vi "Collect Data2D.vi"(8 "error in (no error)":errorcluster, 10 "Data2D in":refnum<class "Data2D.lvclass">, 11 "AbstractCollector2D in":refnum<class "AbstractCollector2D.lvclass">) -> (0 "error out":errorcluster, 2 "finished?":bool=TRUE, 3 "AbstractCollector2D out":refnum<class "AbstractCollector2D.lvclass">)   [LabVIEW 2014, in "AbstractCollector2D.lvclass"]
uses:
  AbstractCollector2D.lvclass
  Model/Data/Data2D/Data2D.lvclass
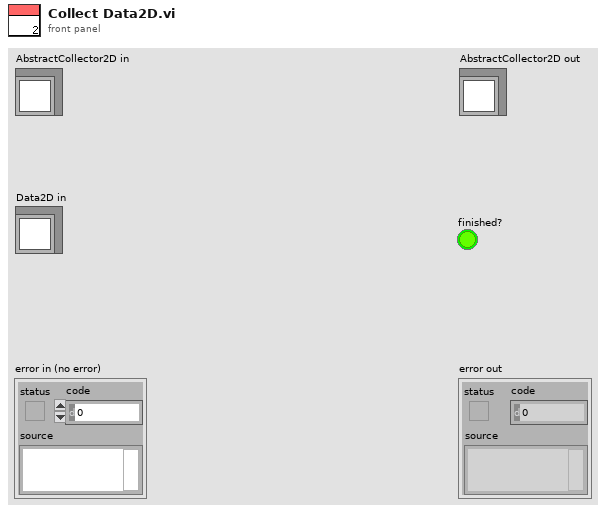
[diagram p1: front panel]
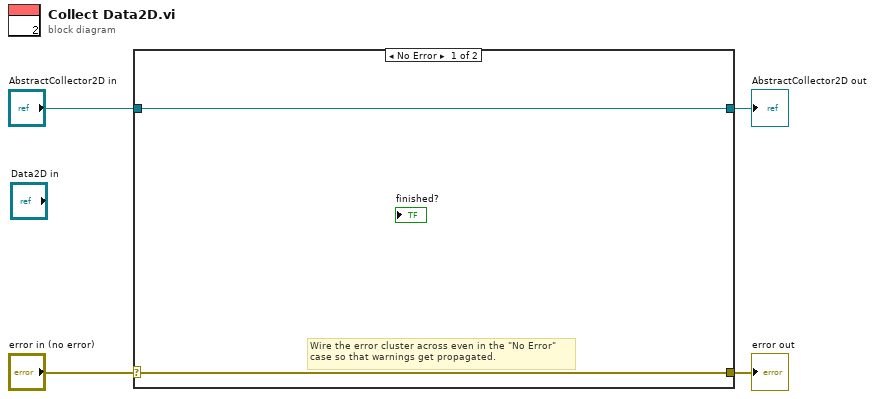
[diagram p0: block diagram]
diagram:
  n1 = case shown="No Error" "error in (no error)" {
    selector: "error in (no error)" -> [w5 w8]
    tunnel: [w5 w8] -> w3
    tunnel: [w6 w7] -> w1
    tunnel: "AbstractCollector2D in" -> [w6 w7]
    frame No Error {
      # "Wire the error cluster across even in the \"No Error\"\ncase so that warnings get propagated."
    }
    frame Error {
    }
  }
  "error out" <- w3
  "AbstractCollector2D out" <- w1
